vi "elevatorCAN.vi"   [LabVIEW 2014]
uses:
  Robot Global Data.vi
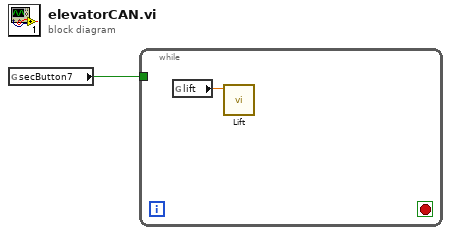
[diagram p0: block diagram]
diagram:
  n1 = global read "Robot Global Data.vi" "secButton7"() -> (w1:bool)
  n2 = while {
    tunnel: w1 -> [_]
    stop <- _ stop-if-true
    n3 = global read "Robot Global Data.vi" "lift"() -> (w2:dbl)
    n4 = call "Lift.vi"("Power Value"=w2) -> ()  [unwired: 11 in]
  }
